vi "simx Create Buffer.vi"(8 "error in (no error)":errorcluster, 11 "bufferSize":i32) -> (0 "error out":errorcluster, 3 "function return":string)   [LabVIEW 2019, in "PXL_V-REP.lvlib"]
doc: "EXTAPI_DLLEXPORT simxUChar* simxCreateBuffer(simxInt bufferSize);"
uses:
  PXL_V-REP.lvlib
  <userlib>/V-REP/remoteApi.dll
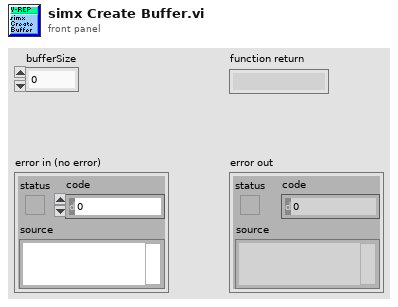
[diagram p1: front panel]
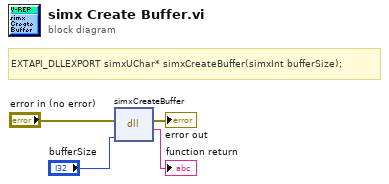
[diagram p0: block diagram]
diagram:
  # "EXTAPI_DLLEXPORT simxUChar* simxCreateBuffer(simxInt bufferSize);"
  n1 = dll-call lib="C:/Program Files (x86)/National Instruments/LabVIEW 2019/user.lib/V-REP/remoteApi.*" fn="simxCreateBuffer"(error in="error in (no error)", "bufferSize"="bufferSize") -> (error out=→"error out":errorcluster, →"function return":string)  [unwired: 3 in, 1 out]
